vi "Get ATM Message.vi"(8 "error in (no error)":errorcluster, 9 "Tokens":cluster{"Name":string, "Value":string}[](array[cluster]), 10 "Message":string, 11 "ATM Messages Ref":refnum<vi>) -> (0 "error out":errorcluster)   [LabVIEW 2020]
doc: "This VI accesses and parses a message string for user display. It provides encapsulation of the core defined messages, so the message set can be updated/modified without having to change this function or any of its callers."
uses:
  Controls/Messages.ctl
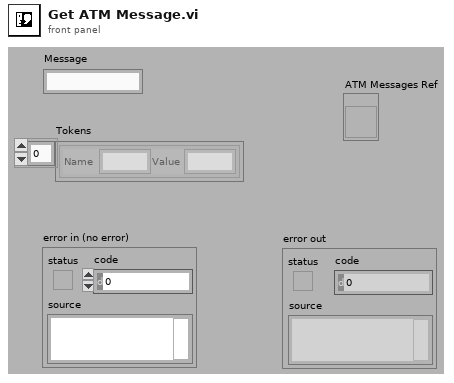
[diagram p1: front panel]
types:
  T1 = typedef "Messages.ctl" = string[][]
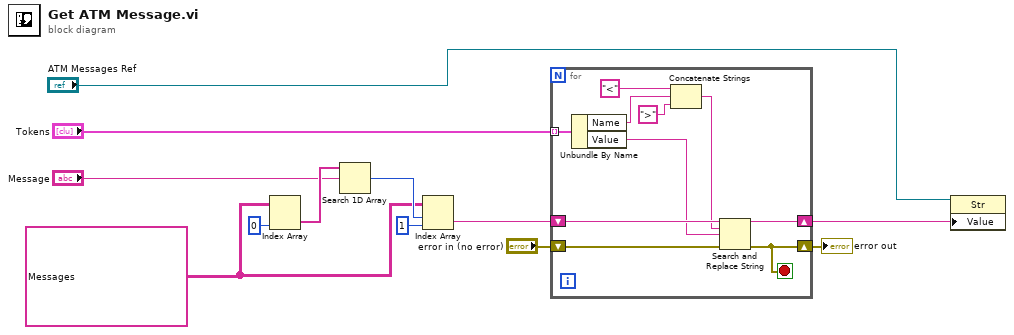
[diagram p0: block diagram]
diagram:
  w3 = T1 [["Welcome", "Welcome to Acme Bank.\nPlease insert your card\nand enter your account\nnumber in the User Input.\n\nPress Enter (E) when done."], ["Main Menu", "Welcome to Acme Bank\n<Name>\n\nPlease select transaction by using the buttons."], ["Account Verification Failed", "Account Information Incorrect.\nPlease Re-Enter Account Number.\nPress Enter (E) when done."], ["Session Terminate", "Your session has been terminated due to inactivity or menu selection.\nPlease take your card.\n\nGoodbye!"], ["Deposit", "Please enter amount to deposit and press Enter (E) when done."], ["Deposit Complete", "$<Amount> Deposited"], ["Withdrawal", "Please enter amount to withdraw and press Enter (E) when done."], ["Withdrawal Complete", "$<Amount> Withdrawn"], ["Withdrawal Failed", "Insufficient funds in account.\nPlease check your balance and try again."], ["Balance Inquiry", "Your Balance Is:\n$<Amount>"]] ("Messages")
  n1 = Index Array(array=w3, index (col)=0 ("disabled index (col)")) -> (element=w11:string[])  [unwired: 1 in]
  n2 = Search 1D Array(1D array=w11, element="Message") -> (index of element=w8:i32)  [unwired: 1 in]
  n3 = Index Array(array=w3, index (row)=w8, index (col)=1 ("disabled index (col)")) -> (element=w6:string)
  n4 = for {
    tunnel: "Tokens" -> [w22] mode=indexing
    shift-right: [w18] -> w5
    shift-left: "error in (no error)" -> [w19]
    shift-right: [w17] -> w2
    shift-left: w6 -> [w21]
    stop <- w18 stop-if-true
    n5 = Unbundle By Name(w22) -> ("Name"=w16:string, "Value"=w20:string)
    n6 = Concatenate Strings("<", w16, ">") -> (w13:string)
    n7 = Search and Replace String(input string=w21, search string=w13, replace string=w20, error in=w19) -> (result string=w17:string, error out=w18:errorcluster)  [unwired: 4 in, 2 out]
  }
  "error out" <- w5
  n8 = property class="Str"(reference="ATM Messages Ref", "Value"=w2) -> ()  [unwired: 1 in, 2 out]
